vi "Stoerungs-Queue in Tabelle Stoermeldepuffer.vi"(9 "Störmeldetexte aus Datei":string[](array[string]), 11 "Queue-Inhalt (FGV Störmeldungen)":T1[](array[typedef])) -> (3 "Tabelle Störmeldungen":string[][](array[string]))   [LabVIEW 2020, in "Stoerungen.lvlib"]
uses:
  Stoerungen.lvlib
  Stoermeldung.ctl
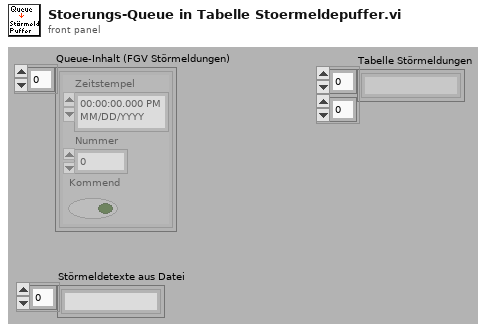
[diagram p1: front panel]
types:
  T1 = typedef "Stoerungen.lvlib/Stoermeldung.ctl" = cluster{"Zeitstempel":timestamp, "Nummer":i32, "Kommend":bool}
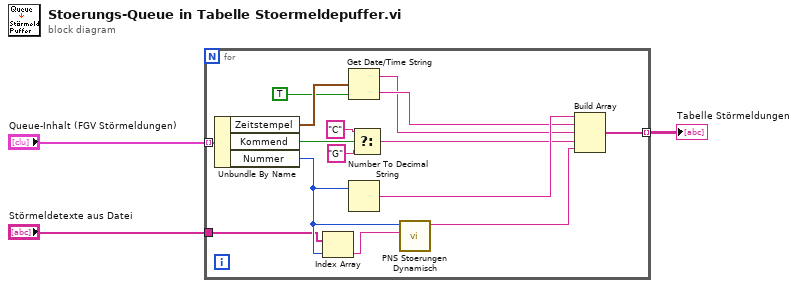
[diagram p0: block diagram]
diagram:
  n1 = for {
    tunnel: "Queue-Inhalt (FGV Störmeldungen)" -> [w18] mode=indexing
    tunnel: "Störmeldetexte aus Datei" -> [w5]
    tunnel: [w8] -> w3 mode=indexing
    n2 = Unbundle By Name(w18) -> ("Zeitstempel"=w17:timestamp, "Kommend"=w12:bool, "Nummer"=w6:i32)
    n3 = Index Array(array=w5, index=w6) -> (element=w4:string)
    n4 = Get Date/Time String(seconds (now)=w17, want seconds? (F)=TRUE ("Angabe von Sekunden? (F)")) -> (date string=w13:string, time string=w14:string)  [unwired: 1 out]
    n5 = Number To Decimal String(number=w6) -> (decimal integer string=w15:string)  [unwired: 1 out]
    n6 = Select(t="C", s=w12, f="G") -> (s? t:f=w9:string)
    n7 = call "PNS Stoerungen Dynamisch.vi"("Störmeldetexte"=w4, "Nummer"=w6) -> ("String"=w7:string)  [unwired: 9 in]
    n8 = Build Array(w15, w14, w13, w9, w7) -> (w8:string[])
  }
  "Tabelle Störmeldungen" <- w3
